vi "Enumerator Reset.vi"(8 "error in (no error)":errorcluster, 11 "List in":refnum<class "DoublyLinkedList.lvclass">) -> (0 "error out":errorcluster, 3 "List out":refnum<class "DoublyLinkedList.lvclass">)   [LabVIEW 2021, in "DoublyLinkedList.lvclass"]
uses:
  DoublyLinkedList.lvclass
  DoublyLinkedList.lvclass/DoublyLinkedList.ctl
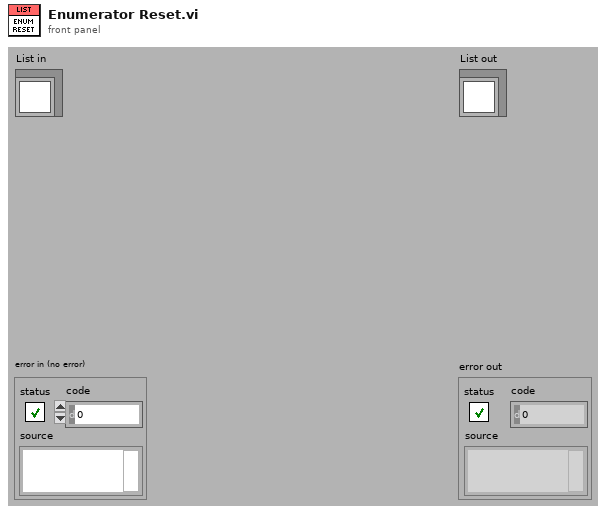
[diagram p1: front panel]
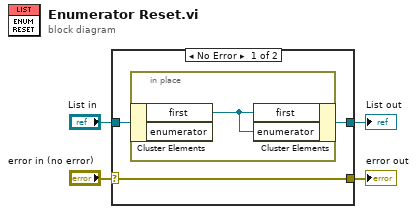
[diagram p0: block diagram]
diagram:
  n1 = case shown="No Error" "error in (no error)" {
    selector: "error in (no error)" -> [w7 w10]
    tunnel: [w7 w10] -> w3
    tunnel: [w5 w9] -> w1
    tunnel: "List in" -> [w6 w9]
    frame No Error {
      n2 = in-place {
        n3 = in-place-cluster #1(w6) -> ("first"=w8:refnum<data-value>)  [unwired: 1 out]
        n4 = in-place-cluster #1("first"=w8, "enumerator"=w8) -> (w5:refnum<class "DoublyLinkedList.lvclass">)
      }
    }
    frame Error {
    }
  }
  "error out" <- w3
  "List out" <- w1
